vi "m1m3_monitorCommand_ApplyAberrationByBendingModes.vi"(8 "error in (no error)":errorcluster, 11 "command_ApplyAberrationByBendingModes_Ctl":T1={"Coefficients[22]"=[0.0, 0.0, 0.0, 0.0, 0.0, 0.0, 0.0, 0.0, 0.0, 0.0, 0.0, 0.0, 0.0, 0.0, 0.0, 0.0, 0.0, 0.0, 0.0, 0.0, 0.0, 0.0]}) -> (0 "error out":errorcluster, 2 "function return":i32, 3 "command_ApplyAberrationByBendingModes_Ctl out":T1)   [LabVIEW 2016, in "SALLV_m1m3.lvlib"]
doc: "int m1m3_shm_monitorCommand_ApplyAberrationByBendingModesLV(m1m3_command_ApplyAberrationByBendingModesLV *command_ApplyAberrationByBendingModes_Ctl );"
uses:
  SALLV_m1m3.lvlib
  DataTypes/command_ApplyAberrationByBendingModes.ctl
  SALLV_m1m3.so
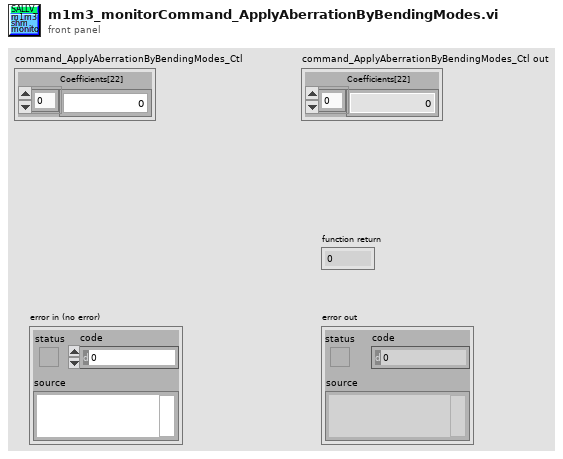
[diagram p1: front panel]
types:
  T1 = typedef "SALLV_m1m3.lvlib/command_ApplyAberrationByBendingModes.ctl" = cluster{"Coefficients[22]":dbl[]}
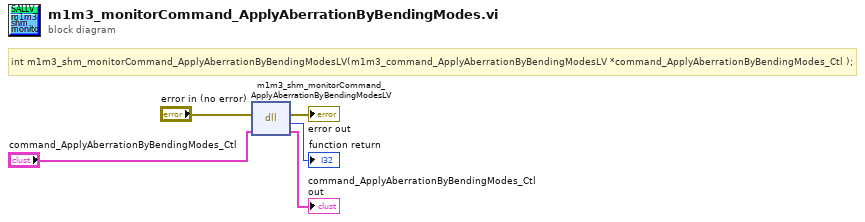
[diagram p0: block diagram]
diagram:
  # "int m1m3_shm_monitorCommand_ApplyAberrationByBendingModesLV(m1m3_command_ApplyAberrationByBendingModesLV *command_ApplyAberrationByBendingModes_Ctl );"
  n1 = dll-call lib="opt/CODE/SALLV_m1m3/SALLV_m1m3.*" fn="m1m3_shm_monitorCommand_ApplyAberrationByBendingModesLV"(error in="error in (no error)", "command_ApplyAberrationByBendingModes_Ctl"="command_ApplyAberrationByBendingModes_Ctl") -> (error out=→"error out":errorcluster, →"function return":i32, "command_ApplyAberrationByBendingModes_Ctl"=→"command_ApplyAberrationByBendingModes_Ctl out":T1)  [unwired: 2 in, 1 out]
